vi "Array API test.vi"() -> ()   [LabVIEW 2013, in "Tagbus PID Module tests.lvlib"]
uses:
  Tagbus PID Module tests.lvlib
  editor node/PID array element.ctl
  editor node/PID Module editor node.lvclass
  module/configuration/PID Module configuration.lvclass
panel:
  in  "Array":T1[](array[typedef])
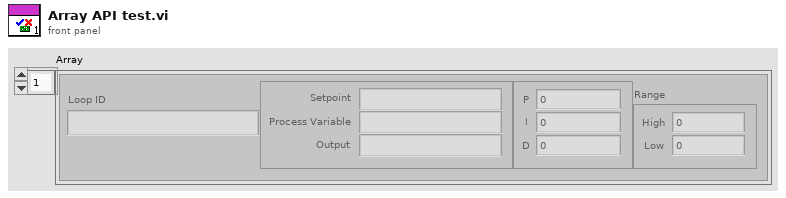
[diagram p1: front panel]
types:
  T1 = typedef "PID Module configuration.lvclass/PID array element.ctl" = cluster{"Loop ID":string, "Tags":cluster{"Setpoint":string, "Process Variable":string, "Output":string}, "Gains":cluster{"P":dbl, "I":dbl, "D":dbl}, "Range":cluster{"High":dbl, "Low":dbl}}
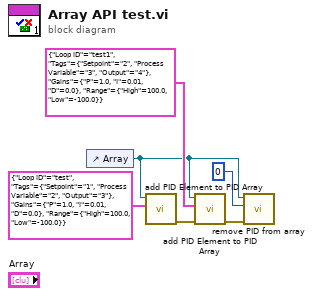
[diagram p0: block diagram]
diagram:
  n1 = control-ref of="Array"() -> (w3:refnum<vi>)
  n2 = call "add PID Element to PID Array.vi"("PID Element"=T1 {"Loop ID"="test", "Tags"={"Setpoint"="1", "Process Variable"="2", "Output"="3"}, "Gains"={"P"=1.0, "I"=0.01, "D"=0.0}, "Range"={"High"=100.0, "Low"=-100.0}}, "PID Array ref in"=w3) -> ("error out"=w5:errorcluster)  [unwired: 9 in]
  n3 = call "add PID Element to PID Array.vi"("error in"=w5, "PID Element"=T1 {"Loop ID"="test1", "Tags"={"Setpoint"="2", "Process Variable"="3", "Output"="4"}, "Gains"={"P"=1.0, "I"=0.01, "D"=0.0}, "Range"={"High"=100.0, "Low"=-100.0}}, "PID Array ref in"=w3) -> ("error out"=w2:errorcluster)  [unwired: 8 in]
  n4 = call "remove PID from array.vi"("error in"=w2, "line number"=0, "operations table"=w3) -> ()  [unwired: 8 in, 1 out]
